vi "JSON FASES.vi"(7 "time":u32, 8 "error in":errorcluster, 9 "Fase":u32, 10 "Corriente":dbl, 11 "Potencia":dbl) -> (0 "error out":errorcluster, 3 "JSON Object out":refnum<class "JSON Object.lvclass">)   [LabVIEW 2015]
uses:
  <vilib>/addons/JSON API/JSON Scalar/Set SGL.vi
  <vilib>/addons/JSON API/JSON Object/Set Object Item by name.vi
  <vilib>/addons/JSON API/JSON Scalar/Set U32.vi
  <vilib>/addons/JSON API/JSON Object/JSON Object.lvclass
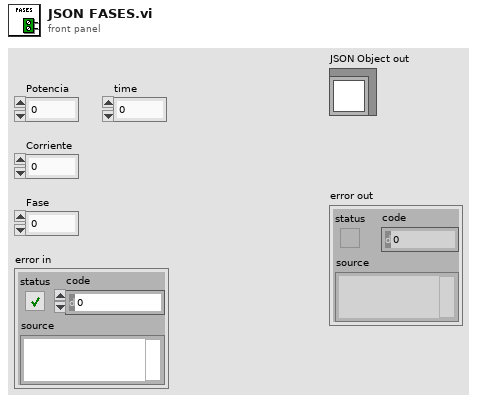
[diagram p1: front panel]
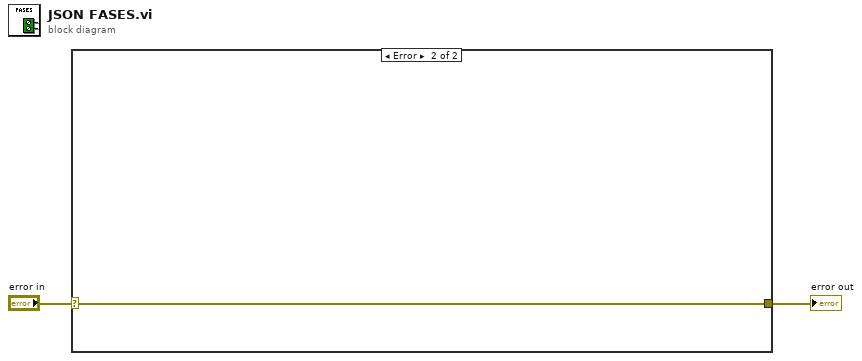
[diagram p0: block diagram]
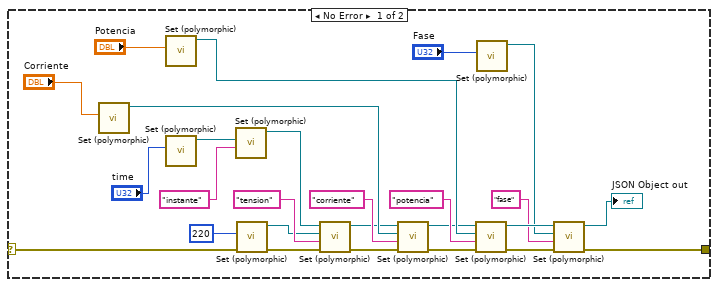
[diagram p2: hidden frame]
diagram:
  n1 = case shown="Error" "error in" {
    selector: "error in" -> [w3 w29]
    tunnel: [w9 w29] -> w2
    frame No Error {
      n2 = call-poly <vilib>:"Set (polymorphic).vi"("Numeric"="Corriente") -> ("JSON Scalar out"=w18:refnum<class "JSON Scalar.lvclass">)  [unwired: 9 in, 1 out]
      n3 = call-poly <vilib>:"Set (polymorphic).vi"("Numeric"="Potencia") -> ("JSON Scalar out"=w21:refnum<class "JSON Scalar.lvclass">)  [unwired: 9 in, 1 out]
      n4 = call-poly <vilib>:"Set (polymorphic).vi"("Numeric"="time") -> ("JSON Scalar out"=w6:refnum<class "JSON Scalar.lvclass">)  [unwired: 9 in, 1 out]
      n5 = call-poly <vilib>:"Set (polymorphic).vi"("name"="instante", "Value"=w6) -> ("JSON Object out"=w4:refnum<class "JSON Object.lvclass">)  [unwired: 7 in, 2 out]
      n6 = call-poly <vilib>:"Set (polymorphic).vi"("error in (no error)"=w3, "Numeric"=u32 220) -> ("error out"=w13:errorcluster, "JSON Scalar out"=w11:refnum<class "JSON Scalar.lvclass">)  [unwired: 8 in]
      n7 = call-poly <vilib>:"Set (polymorphic).vi"("error in (no error)"=w13, "name"="tension", "Value"=w11, "JSON Object in"=w4) -> ("error out"=w17:errorcluster, "JSON Object out"=w15:refnum<class "JSON Object.lvclass">)  [unwired: 5 in, 1 out]
      n8 = call-poly <vilib>:"Set (polymorphic).vi"("error in (no error)"=w17, "name"="corriente", "Value"=w18, "JSON Object in"=w15) -> ("error out"=w27:errorcluster, "JSON Object out"=w19:refnum<class "JSON Object.lvclass">)  [unwired: 5 in, 1 out]
      n9 = call-poly <vilib>:"Set (polymorphic).vi"("error in (no error)"=w27, "name"="potencia", "Value"=w21, "JSON Object in"=w19) -> ("error out"=w28:errorcluster, "JSON Object out"=w26:refnum<class "JSON Object.lvclass">)  [unwired: 5 in, 1 out]
      n10 = call-poly <vilib>:"Set (polymorphic).vi"("Numeric"="Fase") -> ("JSON Scalar out"=w25:refnum<class "JSON Scalar.lvclass">)  [unwired: 9 in, 1 out]
      n11 = call-poly <vilib>:"Set (polymorphic).vi"("error in (no error)"=w28, "name"="fase", "Value"=w25, "JSON Object in"=w26) -> ("error out"=w9:errorcluster, "JSON Object out"=→"JSON Object out":refnum<class "JSON Object.lvclass">)  [unwired: 5 in, 1 out]
    }
    frame Error {
    }
  }
  "error out" <- w2
